vi "Actor Core.vi"(8 "error in":errorcluster, 11 "Nested in":refnum<class "Calling Actor.lvclass">) -> (0 "error out":errorcluster, 3 "Actor out":refnum<class "Actor.lvclass">)   [LabVIEW 2018, in "Calling Actor.lvlib" / "Calling Actor.lvclass"]
doc: "(<B>Filename</B>: Actor Framework.lvlib:Actor.lvclass:Actor Core.vi)\n\nReceives messages to the actor, reacts to them, and initiates any error handling that may shut the actor down.\n\nDescendant classes may override this VI to append parallel tasks for the actor to complete while it handles messages. Overrides use the Call Parent Method node."
uses:
  Calling Actor.lvclass
  C:/Program Files (x86)/National Instruments/LabVIEW 2018/vi.lib/ActorFramework/Actor/Actor.lvclass
  <vilib>/ActorFramework/Actor/Actor.lvclass
  Nested Actor/Nested Actor.lvclass
  Calling Actor Messages/Update UI Msg/Update UI Msg.lvclass
  F:/Gitlab Repository/LabVIEW-Study/9.Abstract Messages in LabVIEW Framework/Corrent Action/Nested Actor Messages/New Data Msg/New Data Msg.lvclass
  Nested Actor/Nested Actor.lvclass/Nested Actor.ctl
  <vilib>/ActorFramework/Actor/Actor.lvclass/Actor.ctl
  <vilib>/ActorFramework/Message Enqueuer/Message Enqueuer.lvclass/Message Enqueuer.ctl
  Calling Actor.lvclass/Calling Actor.ctl
  <vilib>/ActorFramework/Message Enqueuer/Init from Existing Queue.vi
  <vilib>/ActorFramework/Message Enqueuer/Enqueue.vi
  <vilib>/ActorFramework/Stop Msg/Stop Msg.lvclass
  C:/Program Files (x86)/National Instruments/LabVIEW 2018/vi.lib/ActorFramework/Message/Message.lvclass
  <vilib>/ActorFramework/Message Priority Queue/Priority Enqueue.vi
  <vilib>/ActorFramework/Message Enqueuer/Message Enqueuer.lvclass
panel:
  out "Data Received":string
  # "Calling Actor"
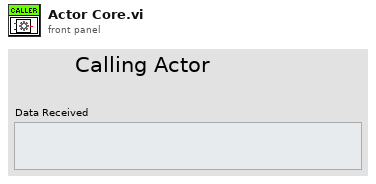
[diagram p1: front panel]
types:
  T1 = cluster{"Stop":refnum<user-event>, "Data Received":refnum<user-event>}
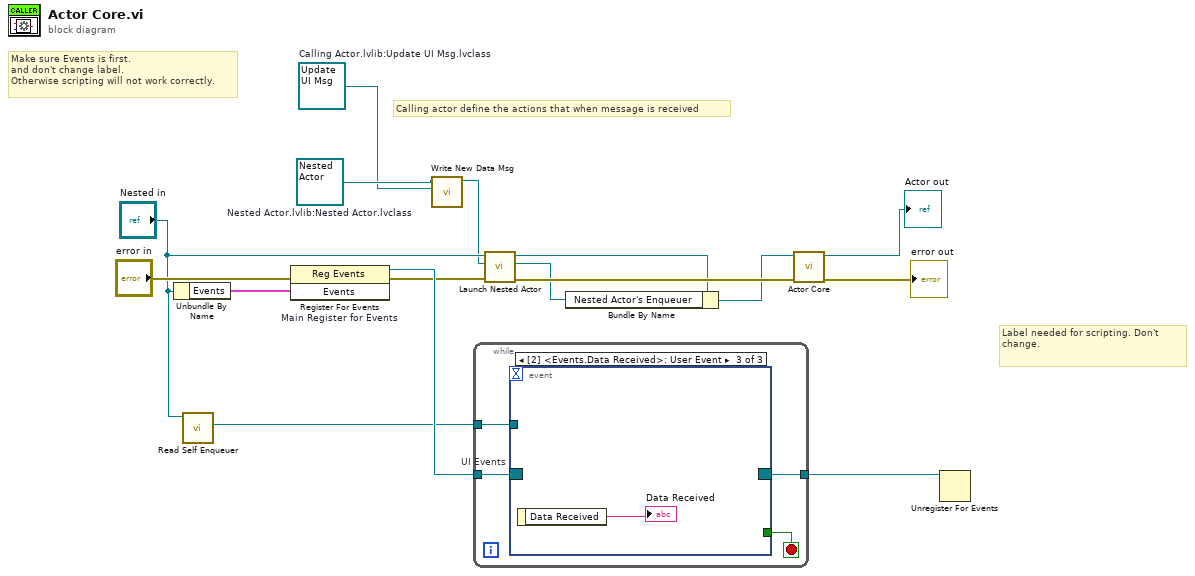
[diagram p0: block diagram]
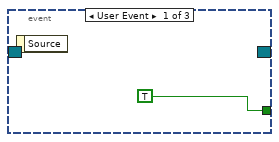
[diagram p2: hidden frame]
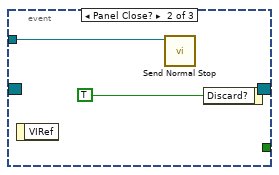
[diagram p3: hidden frame]
diagram:
  w1 = refnum<class "Update UI Msg.lvclass"> refnum  # Calling Actor.lvlib:Update UI Msg.lvclass
  w3 = refnum<class "Nested Actor.lvclass"> refnum  # Nested Actor.lvlib:Nested Actor.lvclass
  # "Calling actor define the actions that when message is received"
  # "Label needed for scripting. Don't change."
  # "Make sure Events is first.\nand don't change label.\nOtherwise scripting will not work correctly."
  n1 = Unbundle By Name("Nested in") -> ("Events"=w13:T1)
  n2 = call <vilib>:"Read Self Enqueuer.vi"("Actor"="Nested in") -> ("Self Enqueuer"=w11:refnum<class "Message Enqueuer.lvclass">)  [unwired: 10 in]
  n3 = register-events "Main Register for Events"(error in="error in", w13) -> (reference out=w14:refnum<event-registration>, error out=w8:errorcluster)  [unwired: 1 in]
  n4 = call "Write New Data Msg.vi"("Nested Actor.lvlib:New Data Msg 2.lvclass"=w1, "Nested Actor in"=w3) -> ("Nested Actor out"=w2:refnum<class "Nested Actor.lvclass">)  [unwired: 9 in]
  n5 = while {
    tunnel: w14 -> [w20]
    tunnel: [w18] -> w12
    tunnel: w11 -> [w17]
    stop <- w19 stop-if-true
    n6 = event "UI Events" shown="[2] <Events.Data Received>: User Event" {
      selector: w20 -> [_ _ _]
      dyn-events: [_ _ _] -> w18
      timeout: _ -> [_ _ _]
      tunnel: [TRUE _ _] -> w19
      tunnel: w17 -> [_ w22 _]
      event User Event {
        n7 = event-data() -> ()  [unwired: 1 in, 1 out]
      }
      event Panel Close? {
        n8 = event-data() -> ()  [unwired: 1 in, 1 out]
        n9 = call <vilib>:"Send Normal Stop.vi"("Message Enqueuer"=w22) -> ()  [unwired: 10 in, 1 out]
        n10 = event-data("Discard?"=TRUE) -> ()  [unwired: 1 in, 1 out]
      }
      event User Event {
        n11 = event-data() -> ("Data Received"=→"Data Received":string)  [unwired: 1 in]
      }
    }
  }
  n12 = call <vilib>:"Launch Nested Actor.vi"("error in (no error)"=w8, "Nested Actor"=w2, "Caller Actor in"="Nested in") -> ("error out"=w7:errorcluster, "Nested Actor's Enqueuer"=w5:refnum<class "Message Enqueuer.lvclass">, "Caller Actor out"=w6:refnum<class "Calling Actor.lvclass">)  [unwired: 6 in]
  n13 = Bundle By Name(cluster=w6, "Nested Actor's Enqueuer"=w5) -> (w4:refnum<class "Calling Actor.lvclass">)
  n14 = call-parent "Actor Core.vi"("error in"=w7, "Actor in"=w4) -> ("error out"=→"error out":errorcluster, "Actor out"=→"Actor out":refnum<class "Actor.lvclass">)  [unwired: 8 in]
  n15 = Unregister For Events(event registration refnum=w12) -> ()  [unwired: 1 in, 1 out]
